vi "BiaxXsig process.vi"(0 "voltage data":dbl[](array[numeric]) format="%.2f", 2 "Numeric":i32=4, 5 "error in (no error)":errorcluster) -> (6 "signal to file (Volt)":sgl[](array[numeric]) format="%.2f", 7 "AUX8":dbl format="%.2f", 8 "AUX7":dbl format="%.2f", 9 "AUX6":dbl format="%.2f", 10 "AUX5":dbl format="%.2f", 11 "error out":errorcluster, 12 "Hor LVDT":dbl format="%.2f", 13 "AUX4":dbl format="%.2f", 14 "Hor Load":dbl format="%.2f", 15 "Vert Load":dbl format="%.2f", 16 "Vert LVDT":dbl format="%.2f", 17 "AUX1":dbl format="%.2f", 18 "AUX2":dbl format="%.2f", 19 "AUX3":dbl format="%.2f")   [LabVIEW 2013]
doc: "This vi accepts the raw voltage data from the following channels: \nCh 0 = Conf. Press. Amp. (0-5)\nCh 1 = Fluid Press. Amp (0-5)\nCh 2 = Temp. Amp (0-1.25 V)\nCh 3 = Displacement Transducer (-2.5 to +2.5 Volt)The data is acquired and processed one point at a time (a non-buffered acquisition). \nCh 4 = Load cell after amplification. 12600 lbsf/volt \n\nThe voltage data array contains the data that the example VI just retrieved from the buffer, one sample per channel. It is a one-dimensional array, indexed by channel.\n\nThe processed data array is returned to the example VI to be displayed.\n\nError in is a cluster that indicates if an error has occurred. If so, this VI does not try to process the data, it just returns the voltage data and error unchanged. If an error occurs in your data processing, you should set the following values in the error out cluster:\n\n (bool) status: TRUE.\n\n (i32) code: the error code associated with an error.\n A value of 0 means no error, a negative value is an error,\n and a positive value is a warning.\n\n (string) source: an indication of where the \n error occurred, usually the name of the VI."
panel:
  # "Sig. Eng. Units"
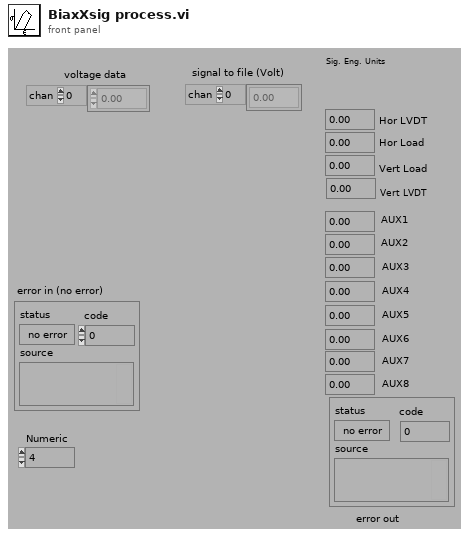
[diagram p1: front panel]
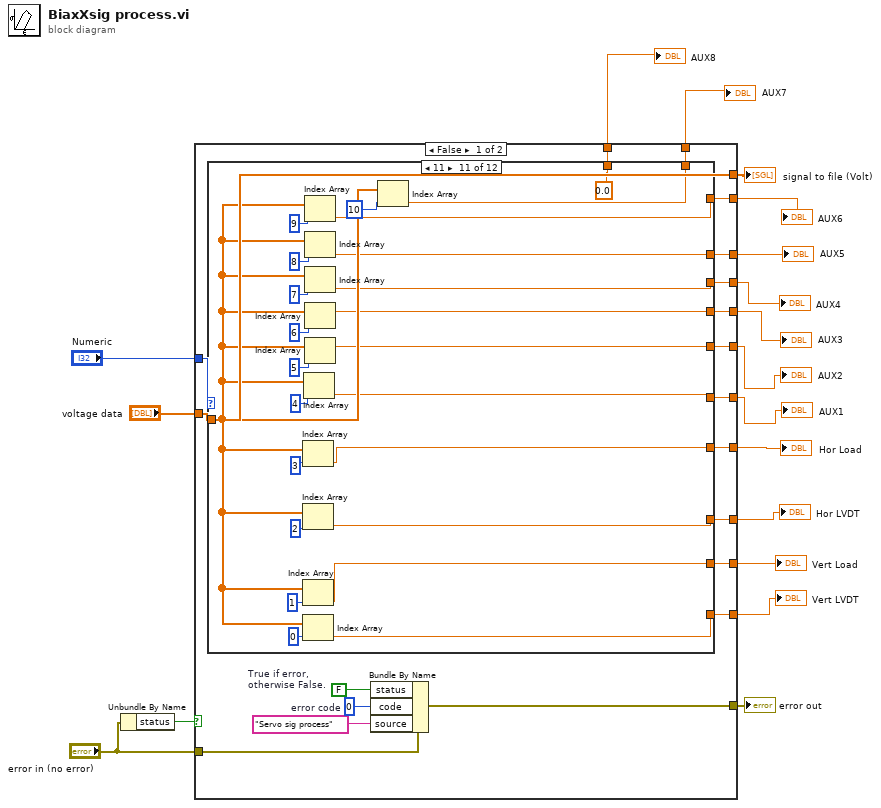
[diagram p0: block diagram]
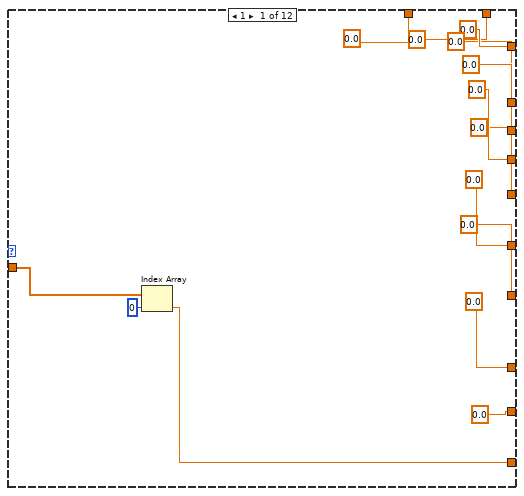
[diagram p2: hidden frame]
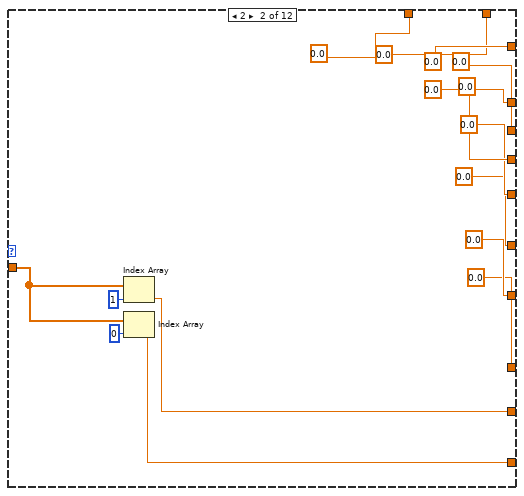
[diagram p3: hidden frame]
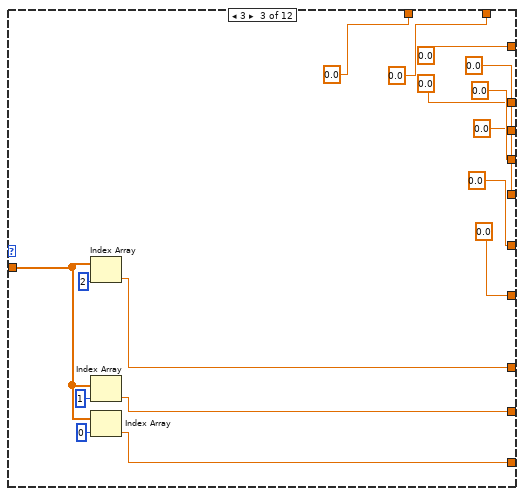
[diagram p4: hidden frame]
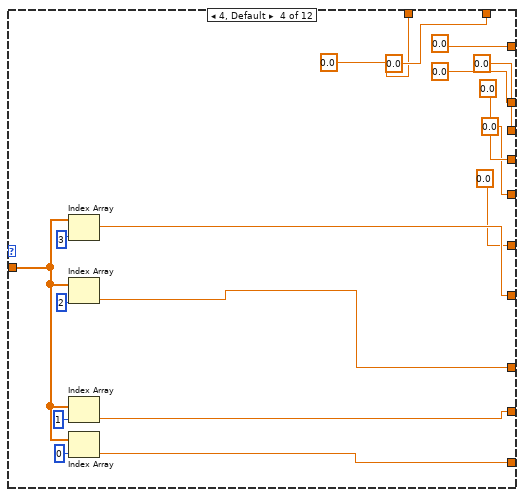
[diagram p5: hidden frame]
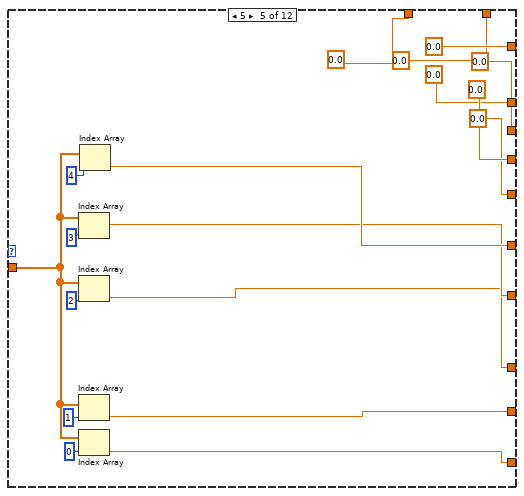
[diagram p6: hidden frame]
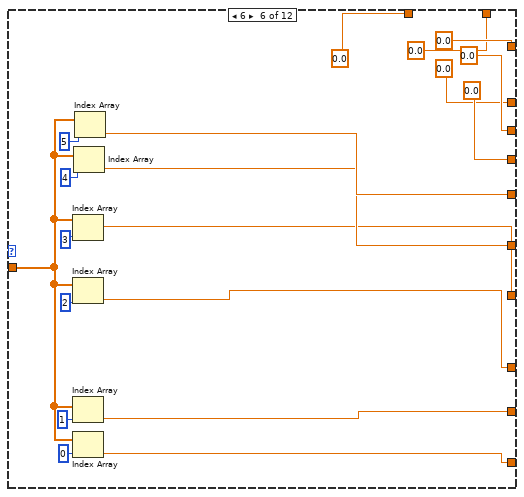
[diagram p7: hidden frame]
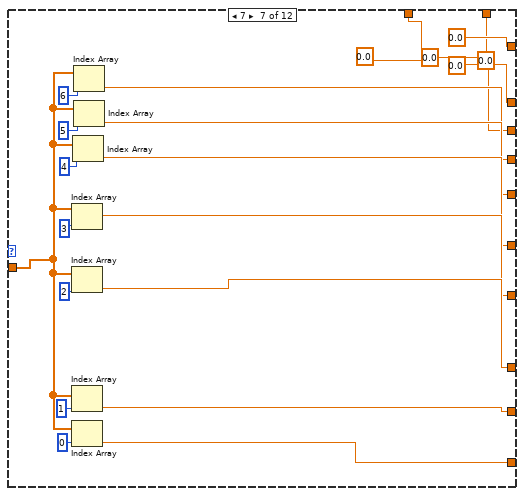
[diagram p8: hidden frame]
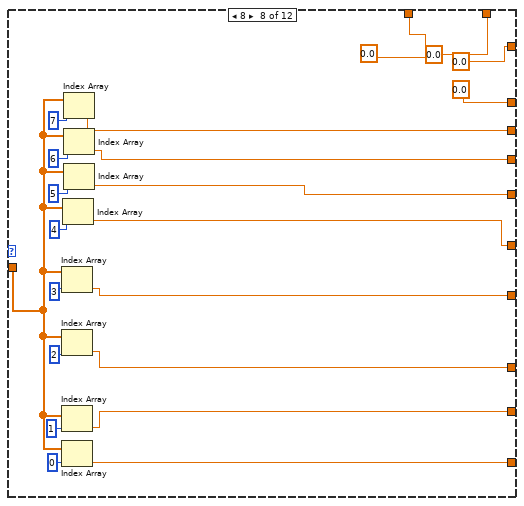
[diagram p9: hidden frame]
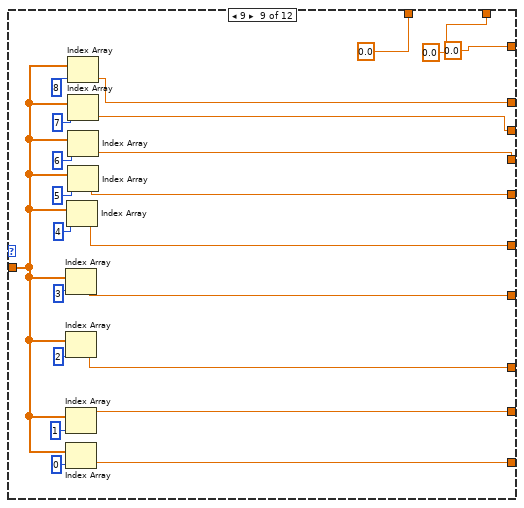
[diagram p10: hidden frame]
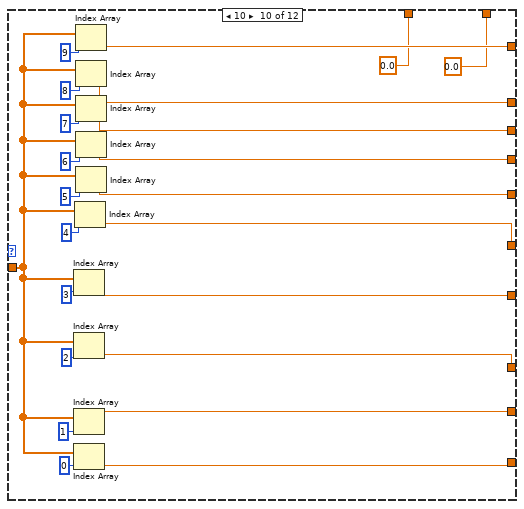
[diagram p11: hidden frame]
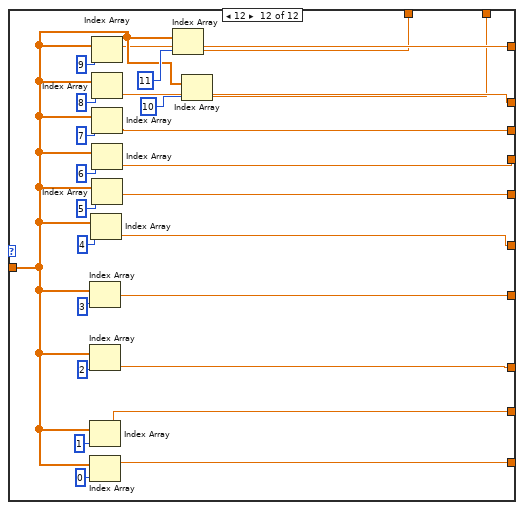
[diagram p12: hidden frame]
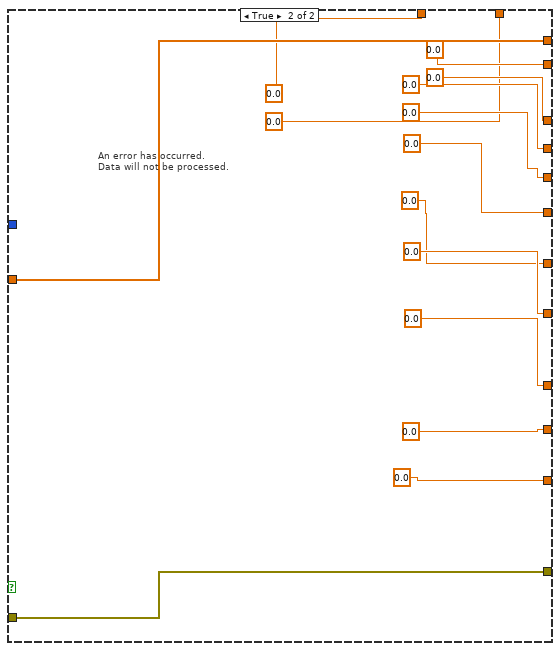
[diagram p13: hidden frame]
diagram:
  n1 = Unbundle By Name("error in (no error)") -> ("status"=w15:bool)
  n2 = case shown="False" w15 {
    tunnel: "error in (no error)" -> [w33 w284]
    tunnel: [w37 w284] -> w18
    tunnel: "voltage data" -> [w32 w285]
    tunnel: [w32 w285] -> w16
    tunnel: "Numeric" -> [w31 _]
    tunnel: [w30 sgl 0.0] -> w5
    tunnel: [w29 sgl 0.0] -> w12
    tunnel: [w28 sgl 0.0] -> w11
    tunnel: [w19 sgl 0.0] -> w10
    tunnel: [w27 sgl 0.0] -> w9
    tunnel: [w26 sgl 0.0] -> w8
    tunnel: [w25 sgl 0.0] -> w7
    tunnel: [w24 sgl 0.0] -> w6
    tunnel: [w22 sgl 0.0] -> w4
    tunnel: [w23 sgl 0.0] -> w3
    tunnel: [w21 sgl 0.0] -> w2
    tunnel: [w20 sgl 0.0] -> w1
    frame False {
      w36 = 0  # error code
      w34 = FALSE  # True if error, otherwise False.
      n3 = case shown="11" w31 {
        tunnel: w32 -> [w50 w64 w79 w95 w112 w130 w149 w169 w182 w202 w235 w259]
        tunnel: [sgl 0.0 sgl 0.0 sgl 0.0 sgl 0.0 sgl 0.0 sgl 0.0 sgl 0.0 w168 w191 w205 w227 w251] -> w30
        tunnel: [sgl 0.0 sgl 0.0 sgl 0.0 sgl 0.0 sgl 0.0 sgl 0.0 w142 w167 w190 w206 w228 w252] -> w29
        tunnel: [sgl 0.0 sgl 0.0 sgl 0.0 sgl 0.0 sgl 0.0 w129 w143 w166 w189 w207 w229 w253] -> w28
        tunnel: [sgl 0.0 sgl 0.0 w78 w92 w109 w126 w146 w165 w186 w210 w232 w256] -> w27
        tunnel: [sgl 0.0 w63 w77 w93 w108 w125 w147 w164 w185 w211 w233 w257] -> w26
        tunnel: [w49 w62 w76 w94 w107 w124 w148 w163 w184 w212 w234 w258] -> w25
        tunnel: [sgl 0.0 sgl 0.0 sgl 0.0 sgl 0.0 w111 w128 w144 w162 w188 w208 w230 w254] -> w24
        tunnel: [sgl 0.0 sgl 0.0 sgl 0.0 sgl 0.0 sgl 0.0 sgl 0.0 sgl 0.0 sgl 0.0 sgl 0.0 w203 w225 w249] -> w23
        tunnel: [sgl 0.0 sgl 0.0 sgl 0.0 sgl 0.0 sgl 0.0 sgl 0.0 sgl 0.0 sgl 0.0 w181 w204 w226 w250] -> w22
        tunnel: [sgl 0.0 sgl 0.0 sgl 0.0 sgl 0.0 sgl 0.0 sgl 0.0 sgl 0.0 sgl 0.0 sgl 0.0 sgl 0.0 w224 w248] -> w21
        tunnel: [sgl 0.0 sgl 0.0 sgl 0.0 sgl 0.0 sgl 0.0 sgl 0.0 sgl 0.0 sgl 0.0 sgl 0.0 sgl 0.0 sgl 0.0 w247] -> w20
        tunnel: [sgl 0.0 sgl 0.0 sgl 0.0 w91 w110 w127 w145 w161 w187 w209 w231 w255] -> w19
        frame 1 {
          n4 = Index Array(array=w50, index=0) -> (element=w49:dbl)
        }
        frame 2 {
          n5 = Index Array(array=w64, index=1) -> (element=w63:dbl)
          n6 = Index Array(array=w64, index=0) -> (element=w62:dbl)
        }
        frame 3 {
          n7 = Index Array(array=w79, index=2) -> (element=w78:dbl)
          n8 = Index Array(array=w79, index=1) -> (element=w77:dbl)
          n9 = Index Array(array=w79, index=0) -> (element=w76:dbl)
        }
        frame 4, Default {
          n10 = Index Array(array=w95, index=3) -> (element=w91:dbl)
          n11 = Index Array(array=w95, index=2) -> (element=w92:dbl)
          n12 = Index Array(array=w95, index=1) -> (element=w93:dbl)
          n13 = Index Array(array=w95, index=0) -> (element=w94:dbl)
        }
        frame 5 {
          n14 = Index Array(array=w112, index=3) -> (element=w110:dbl)
          n15 = Index Array(array=w112, index=2) -> (element=w109:dbl)
          n16 = Index Array(array=w112, index=1) -> (element=w108:dbl)
          n17 = Index Array(array=w112, index=0) -> (element=w107:dbl)
          n18 = Index Array(array=w112, index=4) -> (element=w111:dbl)
        }
        frame 6 {
          n19 = Index Array(array=w130, index=3) -> (element=w127:dbl)
          n20 = Index Array(array=w130, index=2) -> (element=w126:dbl)
          n21 = Index Array(array=w130, index=1) -> (element=w125:dbl)
          n22 = Index Array(array=w130, index=0) -> (element=w124:dbl)
          n23 = Index Array(array=w130, index=4) -> (element=w128:dbl)
          n24 = Index Array(array=w130, index=5) -> (element=w129:dbl)
        }
        frame 7 {
          n25 = Index Array(array=w149, index=3) -> (element=w145:dbl)
          n26 = Index Array(array=w149, index=2) -> (element=w146:dbl)
          n27 = Index Array(array=w149, index=1) -> (element=w147:dbl)
          n28 = Index Array(array=w149, index=0) -> (element=w148:dbl)
          n29 = Index Array(array=w149, index=4) -> (element=w144:dbl)
          n30 = Index Array(array=w149, index=6) -> (element=w142:dbl)
          n31 = Index Array(array=w149, index=5) -> (element=w143:dbl)
        }
        frame 8 {
          n32 = Index Array(array=w169, index=3) -> (element=w161:dbl)
          n33 = Index Array(array=w169, index=2) -> (element=w165:dbl)
          n34 = Index Array(array=w169, index=1) -> (element=w164:dbl)
          n35 = Index Array(array=w169, index=0) -> (element=w163:dbl)
          n36 = Index Array(array=w169, index=4) -> (element=w162:dbl)
          n37 = Index Array(array=w169, index=7) -> (element=w168:dbl)
          n38 = Index Array(array=w169, index=6) -> (element=w167:dbl)
          n39 = Index Array(array=w169, index=5) -> (element=w166:dbl)
        }
        frame 9 {
          n40 = Index Array(array=w182, index=3) -> (element=w187:dbl)
          n41 = Index Array(array=w182, index=2) -> (element=w186:dbl)
          n42 = Index Array(array=w182, index=1) -> (element=w185:dbl)
          n43 = Index Array(array=w182, index=0) -> (element=w184:dbl)
          n44 = Index Array(array=w182, index=4) -> (element=w188:dbl)
          n45 = Index Array(array=w182, index=8) -> (element=w181:dbl)
          n46 = Index Array(array=w182, index=7) -> (element=w191:dbl)
          n47 = Index Array(array=w182, index=6) -> (element=w190:dbl)
          n48 = Index Array(array=w182, index=5) -> (element=w189:dbl)
        }
        frame 10 {
          n49 = Index Array(array=w202, index=3) -> (element=w209:dbl)
          n50 = Index Array(array=w202, index=2) -> (element=w210:dbl)
          n51 = Index Array(array=w202, index=1) -> (element=w211:dbl)
          n52 = Index Array(array=w202, index=0) -> (element=w212:dbl)
          n53 = Index Array(array=w202, index=4) -> (element=w208:dbl)
          n54 = Index Array(array=w202, index=9) -> (element=w203:dbl)
          n55 = Index Array(array=w202, index=8) -> (element=w204:dbl)
          n56 = Index Array(array=w202, index=7) -> (element=w205:dbl)
          n57 = Index Array(array=w202, index=6) -> (element=w206:dbl)
          n58 = Index Array(array=w202, index=5) -> (element=w207:dbl)
        }
        frame 11 {
          n59 = Index Array(array=w235, index=3) -> (element=w231:dbl)
          n60 = Index Array(array=w235, index=2) -> (element=w232:dbl)
          n61 = Index Array(array=w235, index=1) -> (element=w233:dbl)
          n62 = Index Array(array=w235, index=0) -> (element=w234:dbl)
          n63 = Index Array(array=w235, index=4) -> (element=w230:dbl)
          n64 = Index Array(array=w235, index=9) -> (element=w225:dbl)
          n65 = Index Array(array=w235, index=8) -> (element=w226:dbl)
          n66 = Index Array(array=w235, index=7) -> (element=w227:dbl)
          n67 = Index Array(array=w235, index=6) -> (element=w228:dbl)
          n68 = Index Array(array=w235, index=5) -> (element=w229:dbl)
          n69 = Index Array(array=w235, index=10) -> (element=w224:dbl)
        }
        frame 12 {
          n70 = Index Array(array=w259, index=3) -> (element=w255:dbl)
          n71 = Index Array(array=w259, index=2) -> (element=w256:dbl)
          n72 = Index Array(array=w259, index=1) -> (element=w257:dbl)
          n73 = Index Array(array=w259, index=0) -> (element=w258:dbl)
          n74 = Index Array(array=w259, index=4) -> (element=w254:dbl)
          n75 = Index Array(array=w259, index=9) -> (element=w249:dbl)
          n76 = Index Array(array=w259, index=8) -> (element=w250:dbl)
          n77 = Index Array(array=w259, index=7) -> (element=w251:dbl)
          n78 = Index Array(array=w259, index=6) -> (element=w252:dbl)
          n79 = Index Array(array=w259, index=5) -> (element=w253:dbl)
          n80 = Index Array(array=w259, index=11) -> (element=w247:dbl)
          n81 = Index Array(array=w259, index=10) -> (element=w248:dbl)
        }
      }
      n82 = Bundle By Name(cluster=w33, "status"=w34, "code"=w36, "source"="Servo sig process") -> (w37:errorcluster)
    }
    frame True {
      # "An error has occurred.\nData will not be processed."
    }
  }
  "signal to file (Volt)" <- w16
  "error out" <- w18
  "Hor LVDT" <- w9
  "Vert Load" <- w8
  "Vert LVDT" <- w7
  "Hor Load" <- w10
  "AUX1" <- w6
  "AUX2" <- w11
  "AUX3" <- w12
  "AUX4" <- w5
  "AUX5" <- w4
  "AUX6" <- w3
  "AUX7" <- w2
  "AUX8" <- w1
